vi "Set Temperature.vi"(6 "Channel":i32, 8 "error in (no error)":errorcluster, 9 "Rate (K/min)":dbl, 10 "Temperature (K)":dbl, 11 "instrument.PPMS in":refnum<class "instrument.PPMS3.lvclass">) -> (0 "error out":errorcluster, 3 "instrument.PPMS out":refnum<class "instrument.PPMS3.lvclass">)   [LabVIEW 2019, in "instrument.PPMS3.lvclass"]
uses:
  instrument.PPMS3.lvclass
  Typedefs/PPMS3.Commands-enum.ctl
  <userlib>/LevyLab/Levylab Instruments/Instrument Types/Cryostat/Typedefs/Set Temperature--cluster.ctl
  e622c359-5744-4b5f-8951-7a0440714a7f.vi
  e622c359-5744-4b5f-8951-7a0440714a7f.vi/586f54ae-3ebd-4873-8cc5-d027b5473104.vi
  <userlib>/LevyLab/Levylab Instruments/SMOs/RemoteControl/API/Remote Client.vi
  <userlib>/LevyLab/Levylab Instruments/Instrument Types/Cryostat/Instrument.Cryostat.lvclass
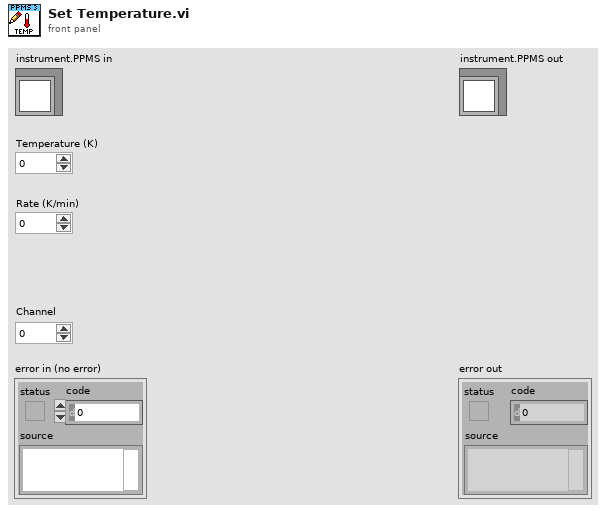
[diagram p1: front panel]
types:
  T1 = typedef "Instrument.Cryostat.lvclass/Set Temperature--cluster.ctl" = cluster{"Temperature (K)":dbl, "Rate (K/min)":dbl, "Channel":i32}
  T2 = typedef "instrument.PPMS3.lvclass/PPMS3.Commands-enum.ctl" = enum16{"Get Magnet Field", "Get Helium Level", "Get Temperature", "Set Magnet Field", "Set Temperature", "getAll"}
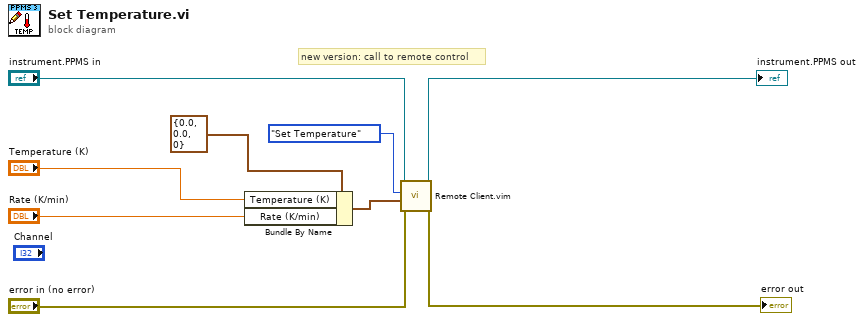
[diagram p0: block diagram]
diagram:
  # "new version: call to remote control"
  n1 = Bundle By Name(cluster=T1 {"Temperature (K)"=0.0, "Rate (K/min)"=0.0, "Channel"=0} ("Set Temperature"), "Temperature (K)"="Temperature (K)", "Rate (K/min)"="Rate (K/min)") -> (w3:T1)
  n2 = call "Remote Client.vim"("error in (no error)"="error in (no error)", "Data"=w3, "Command"=PPMS3.Commands-enum."Set Temperature", "Instrument in"="instrument.PPMS in") -> ("error out"=→"error out":errorcluster, "Instrument out"=→"instrument.PPMS out":refnum<class "instrument.PPMS3.lvclass">)  [unwired: 4 in, 2 out]
